vi "getGridElements.vi"(8 "error in (no error)":errorcluster, 11 "OutcomeList in":refnum<class "GoalList.lvclass">) -> (0 "error out":errorcluster, 2 "Table Interface":string[][](array[string]), 3 "OutcomeList out":refnum<class "GoalList.lvclass">)   [LabVIEW 2020, in "GoalList.lvclass"]
uses:
  GoalList.lvclass
  GoalList.lvclass/GoalList.ctl
  Goal/Goal.lvclass
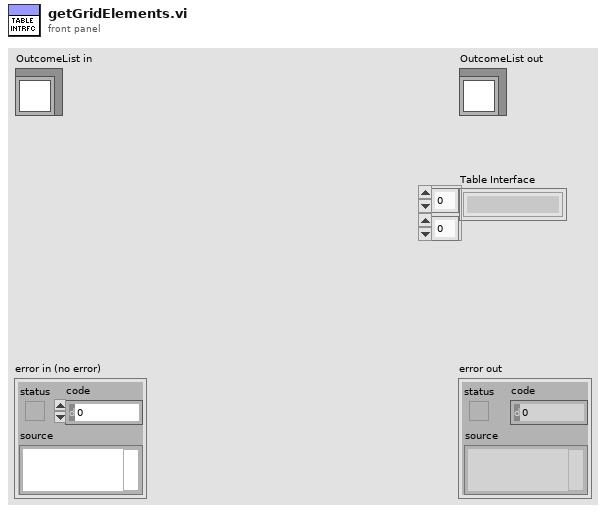
[diagram p1: front panel]
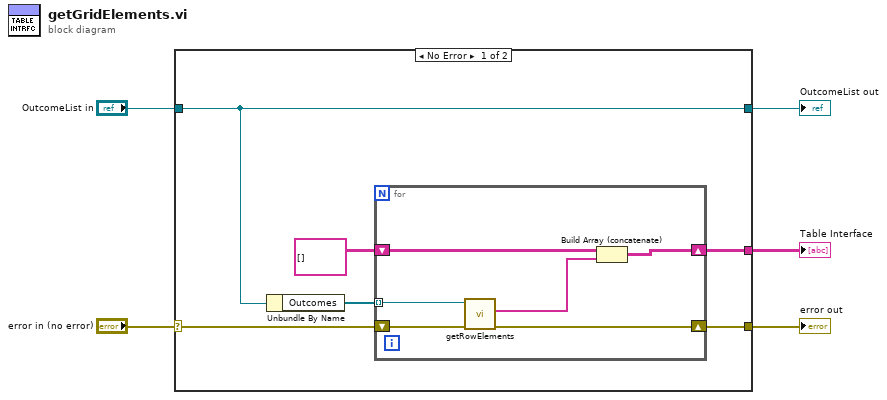
[diagram p0: block diagram]
diagram:
  n1 = case shown="No Error" "error in (no error)" {
    selector: "error in (no error)" -> [w8 w19]
    tunnel: [w7 w19] -> w4
    tunnel: [w11 w18] -> w2
    tunnel: "OutcomeList in" -> [w11 w18]
    tunnel: [w6 _] -> w1
    frame No Error {
      n2 = Unbundle By Name(w11) -> ("Outcomes"=w10:refnum<class "Goal.lvclass">[])
      n3 = for {
        tunnel: w10 -> [w17] mode=indexing
        shift-right: [w14] -> w6
        shift-left: string[][] [] -> [w15]
        shift-right: [w12] -> w7
        shift-left: w8 -> [w16]
        n4 = call-dynamic "getRowElements.vi"("error in (no error)"=w16, "Goal in"=w17) -> ("error out"=w12:errorcluster, "Row Interface"=w13:string[])  [unwired: 7 in, 1 out]
        n5 = Build Array (concatenate)(w15, w13) -> (w14:string[][])
      }
    }
    frame Error {
    }
  }
  "error out" <- w4
  "OutcomeList out" <- w2
  "Table Interface" <- w1
